vi "Begin.vi"() -> (2 "Температура 2":string="25", 3 "Номер образца 2":string="538")   [LabVIEW 2013]
panel:
  out "Ввел 2":bool=TRUE
  out "Boolean 4":bool
  out "Boolean 3":bool
  out "Boolean 2":bool
  out "Boolean":bool
  in  "Ввел":bool
  in  "Т":string="0"
  in  "Номер образца 1":string="0"
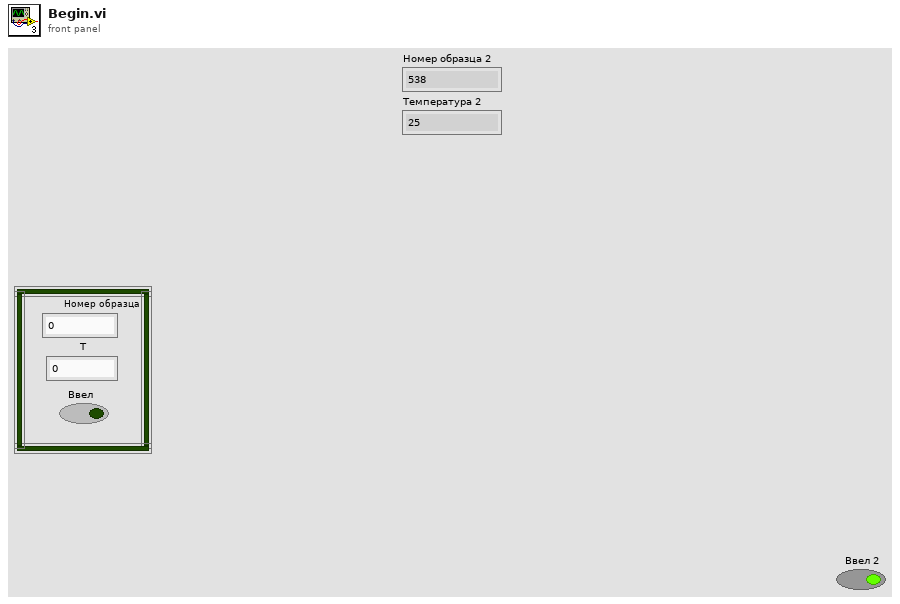
[diagram p1: front panel]
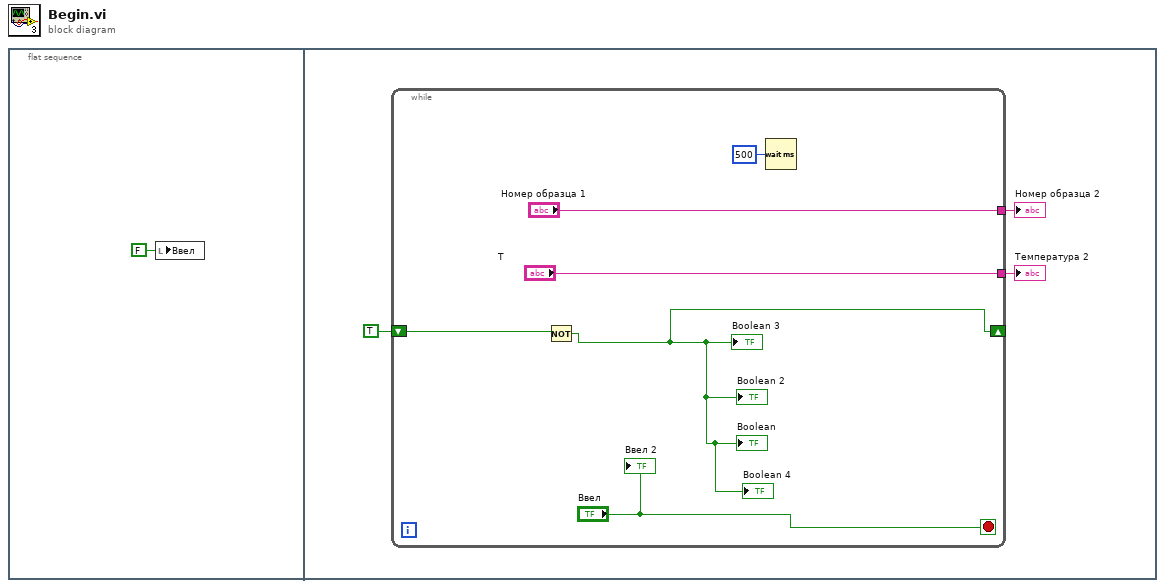
[diagram p0: block diagram]
diagram:
  n1 = flat-sequence {
    frame #0 {
      n2 = local write "Ввел"(FALSE ("Ввел")) -> ()
    }
    frame #1 {
      n3 = while {
        tunnel: ["Номер образца 1"] -> w4
        tunnel: ["Т"] -> w3
        shift-right: [w5] -> _
        shift-left: TRUE -> [w6]
        stop <- "Ввел" stop-if-true
        n4 = Not(x=w6) -> (.not. x?=w5:bool)
        "Boolean 2" <- w5
        "Boolean" <- w5
        "Boolean 4" <- w5
        "Boolean 3" <- w5
        n5 = Wait (ms)(milliseconds to wait=u32 500) -> ()  [unwired: 1 out]
        "Ввел 2" <- "Ввел"
      }
      "Номер образца 2" <- w4
      "Температура 2" <- w3
    }
  }
